vi "DSF.Engine.Execution.Builder.Set RT Thread Parameters.vi"(8 "error in (no error)":errorcluster, 10 "RT Thread Parameters":T1={"Priority"=100, "Processor"=-2}, 11 "Builder in":refnum<class "DSF.Engine.Execution.Builder.lvclass">) -> (0 "error out":errorcluster, 3 "Builder out":refnum<class "DSF.Engine.Execution.Builder.lvclass">)   [LabVIEW 2016, in "DSF.Engine.lvlib" / "DSF.Engine.Execution.Builder.lvclass"]
uses:
  DSF.Engine.Execution.Builder.lvclass
  Shared/Typedefs/DSF.Shared.Typedefs.RT Thread Parameters.ctl
  DSF.Engine.Execution.Builder.lvclass/DSF.Engine.Execution.Builder.ctl
  DSF.Shared.lvlib
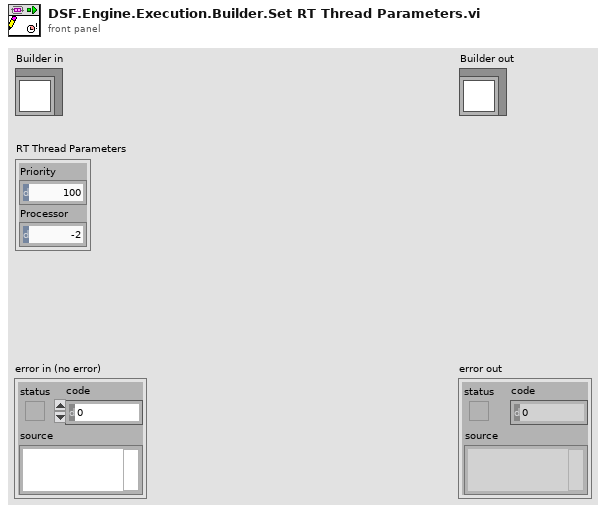
[diagram p1: front panel]
types:
  T1 = typedef "DSF.Shared.lvlib/DSF.Shared.Typedefs.RT Thread Parameters.ctl" = cluster{"Priority":i32, "Processor":i32}
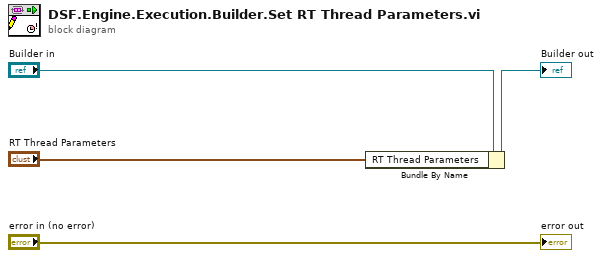
[diagram p0: block diagram]
diagram:
  n1 = Bundle By Name(cluster="Builder in", "RT Thread Parameters"="RT Thread Parameters") -> (→"Builder out":refnum<class "DSF.Engine.Execution.Builder.lvclass">)
  "error out" <- "error in (no error)"
